vi "From HTTP Date String.vi"(11 "HTTP Date String":string) -> (3 "Time Stamp":timestamp)   [LabVIEW 2020, in "HTTP Utils.lvlib"]
uses:
  HTTP Utils.lvlib
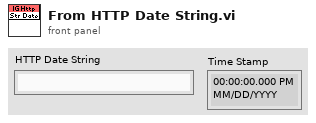
[diagram p1: front panel]
types:
  T1 = typedef "LVDateTimeRec.ctl" = cluster{"fractional second":dbl, "second":i32, "minute":i32, "hour":i32, "day of month":i32, "month":i32, "year":i32, "day of week":i32, "day of year":i32, "DST":i32}
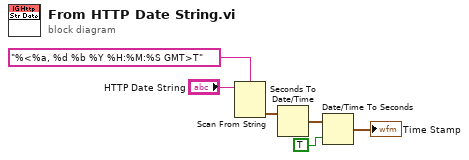
[diagram p0: block diagram]
diagram:
  n1 = Scan From String(format string="%<%a, %d %b %Y %H:%M:%S GMT>T" ("time format string (%c)"), input string="HTTP Date String") -> (output 1=w4:timestamp)  [unwired: 3 in, 3 out]
  n2 = Seconds To Date/Time(time stamp (now)=w4) -> (date time rec=w3:T1)  [unwired: 1 in]
  n3 = Date/Time To Seconds(1:TRUE ("is UTC (F)"), 2:w3) -> (0:→"Time Stamp":timestamp)
